vi "Day 13.2 - Complete Folds.vi"(11 "input":string) -> (2 "output array":bool[][](array[boolean]), 3 "output":i32)   [LabVIEW 2021]
panel:
  out "original array":bool[][](array[boolean])
  out "number":string[](array[string])
  out "Fold":string[](array[string])
  out "dots":i32[][](array[numeric])
  out "Folds":string
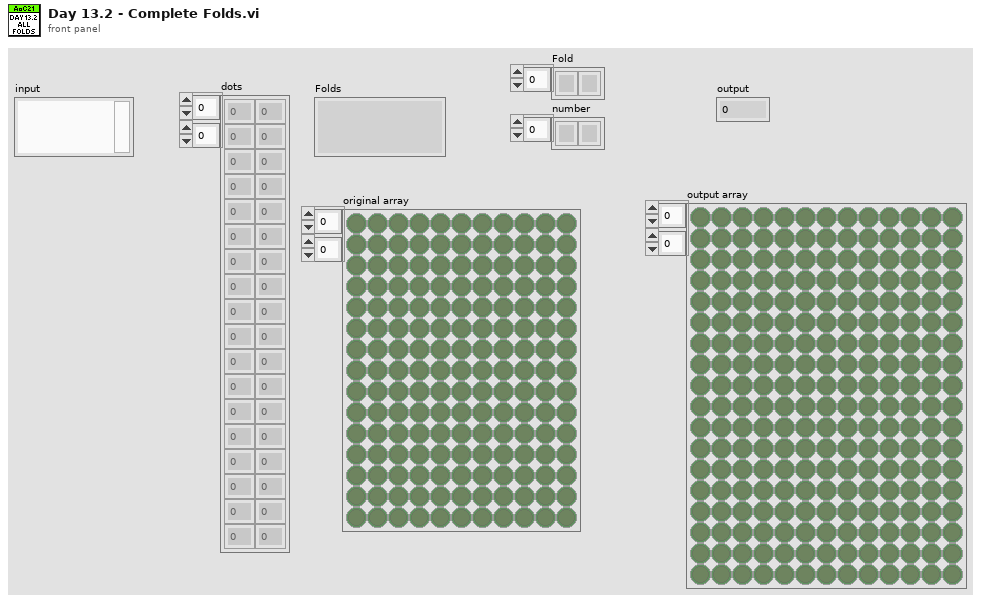
[diagram p1: front panel]
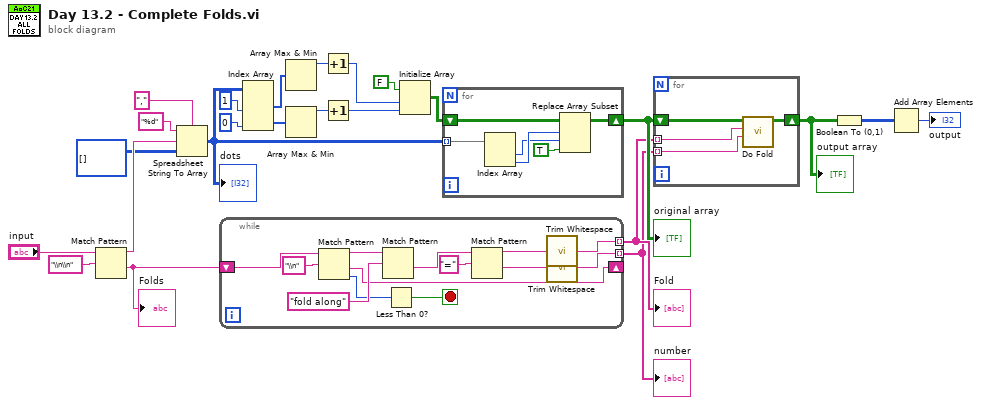
[diagram p0: block diagram]
diagram:
  n1 = Match Pattern(string="input", regular expression="\\n\\n") -> (before substring=w22:string, after substring=w3:string)  [unwired: 1 in, 2 out]
  "Folds" <- w3
  n2 = Spreadsheet String To Array(delimiter (Tab)=",", format string="%d", spreadsheet string=w22, array type (2D Dbl)=i32[][] []) -> (array=w11:i32[][])
  "dots" <- w11
  n3 = while {
    tunnel: [w31] -> w2 mode=indexing
    tunnel: [w30] -> w1 mode=indexing
    shift-right: [w26] -> _
    shift-left: w3 -> [w28]
    stop <- w34 stop-if-true
    n4 = Match Pattern(string=w28, regular expression="\\n") -> (before substring=w27:string, after substring=w26:string, offset past match=w25:i32)  [unwired: 1 in, 1 out]
    n5 = Match Pattern(string=w27, regular expression="fold along") -> (after substring=w36:string)  [unwired: 1 in, 3 out]
    n6 = Less Than 0?(x=w25) -> (x < 0?=w34:bool)
    n7 = Match Pattern(string=w36, regular expression="=") -> (before substring=w33:string, after substring=w32:string)  [unwired: 1 in, 2 out]
    n8 = call <vilib>:"Trim Whitespace.vi"("string"=w33) -> ("trimmed string"=w31:string)  [unwired: 1 in]
    n9 = call <vilib>:"Trim Whitespace.vi"("string"=w32) -> ("trimmed string"=w30:string)  [unwired: 1 in]
  }
  "Fold" <- w2
  "number" <- w1
  n10 = Index Array(array=w11, index (col) #1=1 ("disabled index (col)"), index (col) #2=0 ("index (col)")) -> (element #1=w13:i32[], element #2=w14:i32[])  [unwired: 2 in]
  n11 = Array Max & Min(array=w13) -> (max value=w12:i32)  [unwired: 3 out]
  n12 = Array Max & Min(array=w14) -> (max value=w15:i32)  [unwired: 3 out]
  n13 = Increment(x=w12) -> (x+1=w9:i32)
  n14 = Increment(x=w15) -> (x+1=w8:i32)
  n15 = Initialize Array(FALSE, w9, w8) -> (w10:bool[][])
  n16 = for {
    tunnel: w11 -> [w41] mode=indexing
    shift-right: [w42] -> w7
    shift-left: w10 -> [w43]
    n17 = Index Array(array=w41) -> (element #1=w38:i32, element #2=w39:i32)  [unwired: 2 in]
    n18 = Replace Array Subset(array=w43, new element=TRUE ("new element/subarray"), index (row)=w39, index (col)=w38) -> (w42:bool[][])
  }
  "original array" <- w7
  n19 = for {
    tunnel: w2 -> [w47] mode=indexing
    tunnel: w1 -> [w46] mode=indexing
    shift-right: [w44] -> w6
    shift-left: w7 -> [w45]
    n20 = call "Do Fold.vi"("Fold Line"=w46, "Fold Axis"=w47, "Array in"=w45) -> ("Array out"=w44:bool[][])  [unwired: 8 in]
  }
  "output array" <- w6
  n21 = Boolean To (0,1)(Boolean=w6) -> (0, 1=w5:i16[][])
  n22 = Add Array Elements(numeric array=w5) -> (sum=→"output":i16)
